vi "ProgressPopupWithStatus.vi"(10 "Message":string) -> ()   [LabVIEW 2014, in "hse-ui.lvlib"]
doc: "____\nHAMPEL SOFTWARE ENGINEERING v0.7.0 (2018-07-16 18:12)"
uses:
  hse-ui.lvlib
  ProgressPopupWithStatus_Notifiers.ctl
  FPControl/FPControl_Actions.ctl
panel:
  in  "Deployment Notifiers":T1
  out "Progress String":string="Transferring - This operation may take several minutes."
  in  "Stop":bool
  out "Message out":string
  out "Progress":i8(slide) scale=0.0..100.0
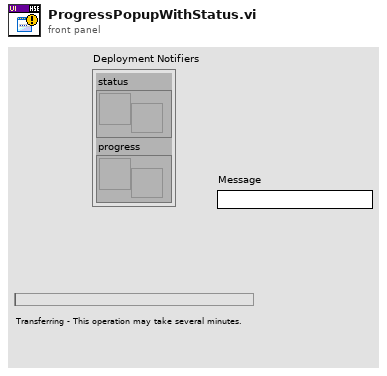
[diagram p1: front panel]
types:
  T1 = typedef "hse-ui.lvlib/ProgressPopupWithStatus_Notifiers.ctl" = cluster{"status":refnum<notifier>, "progress":refnum<notifier>}
  T2 = typedef "hse-ui.lvlib/FPControl_Actions.ctl" = enum16{"Open", "Hide", "Close", "Bring To Front", "Center", "Minimize", "Maximize"}
  T3 = typedef "LVRectTypeDef.ctl" = cluster{"Left":i16, "Top":i16, "Right":i16, "Bottom":i16}
  T4 = cluster{"left":i16, "top":i16, "right":i16, "bottom":i16}
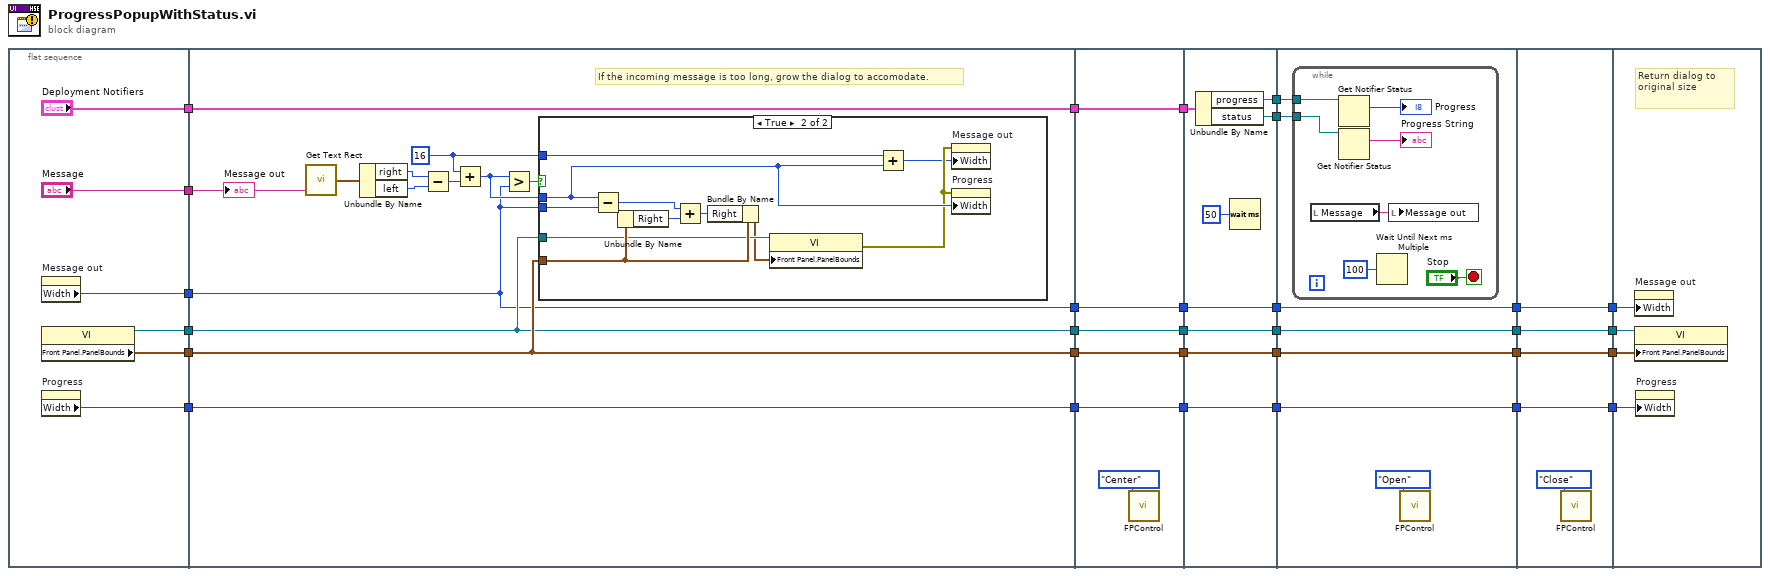
[diagram p0: block diagram]
diagram:
  n1 = flat-sequence {
    tunnel: [w36] -> w6
    tunnel: [w35] -> w5
    tunnel: [w34] -> w4
    tunnel: [w33] -> w3
    tunnel: ["Message"] -> w2
    tunnel: ["Deployment Notifiers"] -> w1
    tunnel: [w39] -> w28
    tunnel: [w40] -> w25
    tunnel: [w41] -> w22
    tunnel: [w42] -> w19
    tunnel: [w37] -> w7
    tunnel: w6 -> [w42]
    tunnel: w5 -> [w41]
    tunnel: w4 -> [w40]
    tunnel: w3 -> [w39]
    tunnel: w2 -> [w38]
    tunnel: w1 -> [w37]
    tunnel: [w66] -> w18
    tunnel: w28 -> [w66]
    tunnel: [w65] -> w16
    tunnel: w25 -> [w65]
    tunnel: [w64] -> w14
    tunnel: w22 -> [w64]
    tunnel: [w63] -> w12
    tunnel: w19 -> [w63]
    tunnel: [w61] -> w8
    tunnel: w7 -> [w61]
    tunnel: w18 -> [w74]
    tunnel: [w74] -> w17
    tunnel: w16 -> [w73]
    tunnel: [w73] -> w15
    tunnel: w14 -> [w72]
    tunnel: [w72] -> w13
    tunnel: w12 -> [w71]
    tunnel: [w71] -> w11
    tunnel: [w69] -> w10
    tunnel: [w68] -> w9
    tunnel: w8 -> [w67]
    tunnel: [w81] -> w29
    tunnel: w17 -> [w81]
    tunnel: [w80] -> w26
    tunnel: w15 -> [w80]
    tunnel: [w79] -> w23
    tunnel: w13 -> [w79]
    tunnel: [w78] -> w20
    tunnel: w11 -> [w78]
    tunnel: w10 -> [w77]
    tunnel: w9 -> [w76]
    tunnel: [w93] -> w30
    tunnel: w29 -> [w93]
    tunnel: [w92] -> w27
    tunnel: w26 -> [w92]
    tunnel: [w91] -> w24
    tunnel: w23 -> [w91]
    tunnel: [w90] -> w21
    tunnel: w20 -> [w90]
    tunnel: w30 -> [w97]
    tunnel: w27 -> [w96]
    tunnel: w24 -> [w95]
    tunnel: w21 -> [w94]
    frame #0 {
      n2 = property on="Message out" class="Str"() -> ("Width"=w33:u32)  [unwired: 2 in, 2 out]
      n3 = property class="VI"() -> (reference out=w34:refnum<vi>, "Front Panel.PanelBounds"=w35:T3)  [unwired: 2 in, 1 out]
      n4 = property on="Progress" class="Slide (strict)"() -> ("Width"=w36:u32)  [unwired: 2 in, 2 out]
    }
    frame #1 {
      w43 = i16 16 ("y")
      # "If the incoming message is too long, grow the dialog to accomodate."
      n5 = call <vilib>:"Get Text Rect.vi"("text"=w38) -> ("rect"=w49:T4)  [unwired: 8 in]
      n6 = Unbundle By Name(w49) -> ("right"=w48:i16, "left"=w47:i16)
      n7 = Subtract(x=w48, y=w47) -> (x-y=w44:i16)
      n8 = Add(x=w43, y=w44) -> (x+y=w46:i16)
      n9 = Greater?(x=w46, y=w39) -> (0:w45:bool)
      n10 = case shown="True" w45 {
        tunnel: w46 -> [_ w60]
        tunnel: w41 -> [_ w59]
        tunnel: w40 -> [_ w58]
        tunnel: w39 -> [_ w57]
        tunnel: w43 -> [_ w50]
        frame False {
        }
        frame True {
          n11 = Subtract(x=w60, y=w57) -> (x-y=w52:u32)
          n12 = Unbundle By Name(w59) -> ("Right"=w53:i16)
          n13 = Add(x=w52, y=w53) -> (x+y=w56:u32)
          n14 = Bundle By Name(cluster=w59, "Right"=w56) -> (w55:T3)
          n15 = property class="VI"(reference=w58, "Front Panel.PanelBounds"=w55) -> (error out=w54:errorcluster)  [unwired: 1 in, 1 out]
          n16 = Add(x=w50, y=w60) -> (x+y=w51:i16)
          n17 = property on="Message out" class="Str"(error in=w54, "Width"=w51) -> ()  [unwired: 1 in, 2 out]
          n18 = property on="Progress" class="Slide (strict)"(error in=w54, "Width"=w60) -> ()  [unwired: 1 in, 2 out]
        }
      }
      "Message out" <- w38
    }
    frame #2 {
      n19 = call "FPControl.vi"("Function"=FPControl_Actions."Center") -> ()  [unwired: 1 in, 10 out]
    }
    frame #3 {
      n20 = Unbundle By Name(w67) -> ("progress"=w69:refnum<notifier>, "status"=w68:refnum<notifier>)
      n21 = Wait (ms)(milliseconds to wait=u32 50) -> ()  [unwired: 1 out]
    }
    frame #4 {
      n22 = while {
        tunnel: w77 -> [w83]
        tunnel: w76 -> [w82]
        stop <- "Stop" stop-if-true
        n23 = local read "Message"() -> (w86:string)
        n24 = Get Notifier Status(notifier=w83) -> (current notification=→"Progress":i8)  [unwired: 1 in, 4 out]
        n25 = Get Notifier Status(notifier=w82) -> (current notification=→"Progress String":string)  [unwired: 1 in, 4 out]
        n26 = Wait Until Next ms Multiple(millisecond multiple=u32 100) -> ()  [unwired: 1 out]
        n27 = local write "Message out"(w86) -> ()
      }
      n28 = call "FPControl.vi"("Function"=FPControl_Actions."Open") -> ()  [unwired: 1 in, 10 out]
    }
    frame #5 {
      n29 = call "FPControl.vi"("Function"=FPControl_Actions."Close") -> ()  [unwired: 1 in, 10 out]
    }
    frame #6 {
      # "Return dialog to original size"
      n30 = property on="Message out" class="Str"("Width"=w97) -> ()  [unwired: 2 in, 2 out]
      n31 = property class="VI"(reference=w96, "Front Panel.PanelBounds"=w95) -> ()  [unwired: 1 in, 2 out]
      n32 = property on="Progress" class="Slide (strict)"("Width"=w94) -> ()  [unwired: 2 in, 2 out]
    }
  }
